vi "MotorenAnsteuern.vi"() -> ()   [LabVIEW 2023]
panel:
  out "IP Adresse":string
  in  "Motor auswählen":string(combo)
  out "Digital":dbl
  out "Drehmoment":dbl
  out "Status/Fehler":dbl
  out "Istgeschwindigkeit":dbl
  out "Handshake":bool
  out "Standby aktiv":bool
  out "Reserviert":bool
  out "SWES inaktiv":bool
  out "Geschwindigkeit erreicht":bool
  out "AS2 aktiv":bool
  out "Warnung":bool
  out "Fehler":bool
  out "in Position":bool
  out "Relativposition übernommen":bool
  out "referenziert":bool
  out "Motor dreht":bool
  out "Bremse geöffnet":bool
  out "Endstufenfreigabe":bool
  out "STO inaktiv":bool
  out "Betriebsbereit":bool
  in  "Stopp":bool
  in  "Digital":dbl
  in  "Deceleration":dbl
  in  "Acceleration":dbl
  in  "Speed":dbl
  in  "Handshake":bool
  in  "Standby":bool
  in  "Inhibit":bool
  in  "Reserviert":bool
  in  "Reservier":bool
  in  "AS2 aktivieren":bool
  in  "Reserviert":bool
  in  "Fehler_Reset":bool
  in  "Start":bool
  in  "Reserviert":bool
  in  "Reserviert":bool
  in  "Reserviert":bool
  in  "Bremse öffnen":bool
  in  "Reserviert":bool
  in  "Enable/ApplicationStop":bool
  in  "Enable/EmergencyStop":bool
  # "zum MOVIDRIVE"
  # "vom MOVIDRIVE"
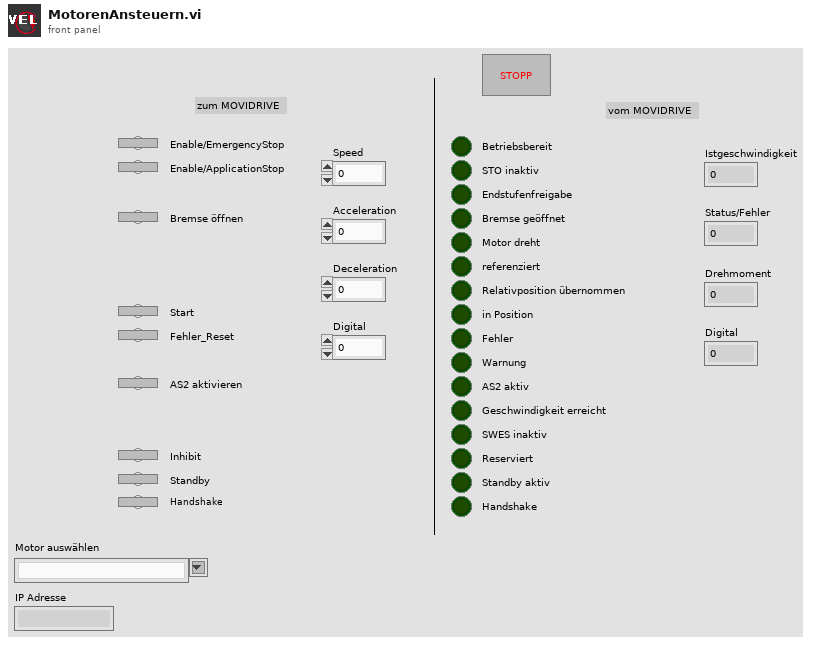
[diagram p1: front panel]
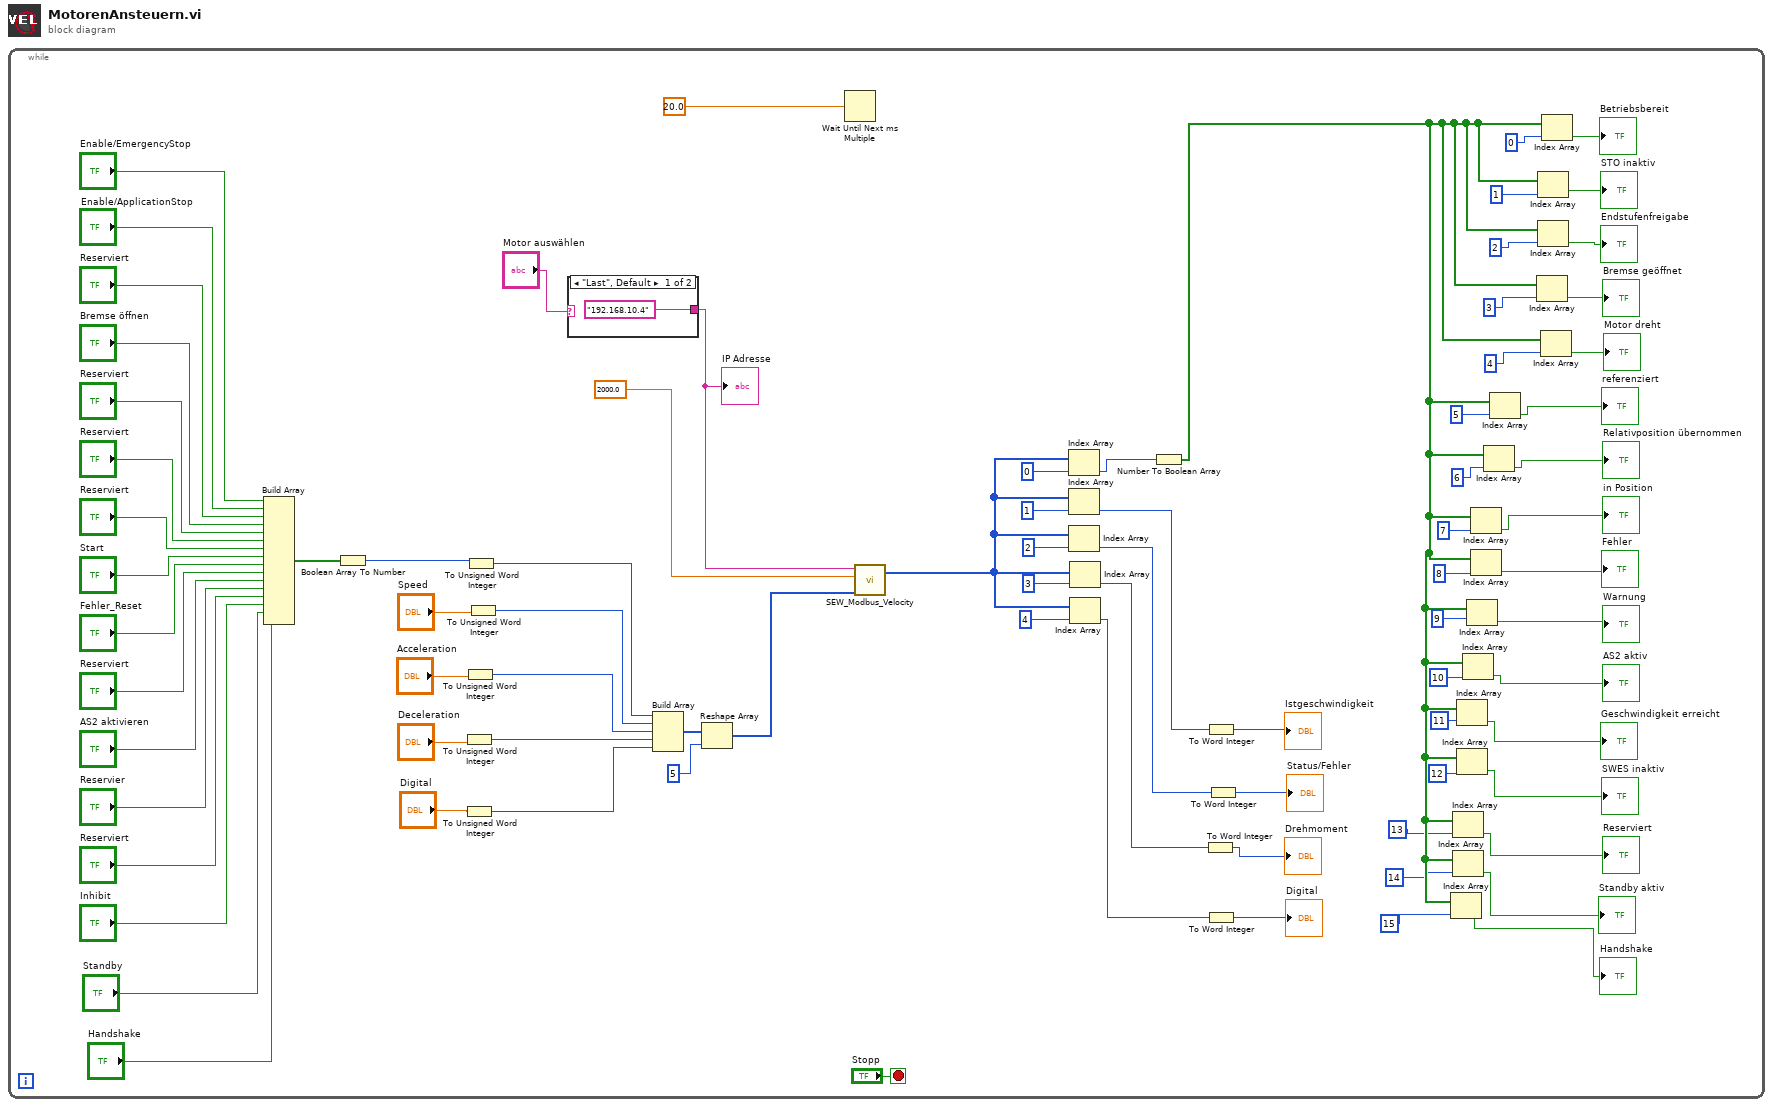
[diagram p0: block diagram]
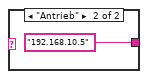
[diagram p2: hidden frame]
diagram:
  n1 = while {
    stop <- "Stopp" stop-if-true
    n2 = Build Array("Enable/EmergencyStop", "Enable/ApplicationStop", "Reserviert", "Bremse öffnen", "Reserviert", "Reserviert", "Reserviert", "Start", "Fehler_Reset", "Reserviert", "AS2 aktivieren", "Reservier", "Reserviert", "Inhibit", "Standby", "Handshake") -> (w71:bool[])
    n3 = Boolean Array To Number(Boolean array=w71) -> (number=w72:u32)
    n4 = To Unsigned Word Integer(number="Deceleration") -> (unsigned 16bit integer=w78:u16)
    n5 = To Unsigned Word Integer(number="Digital") -> (unsigned 16bit integer=w79:u16)
    n6 = To Unsigned Word Integer(number="Acceleration") -> (unsigned 16bit integer=w77:u16)
    n7 = To Unsigned Word Integer(number=w72) -> (unsigned 16bit integer=w76:u16)
    n8 = To Unsigned Word Integer(number="Speed") -> (unsigned 16bit integer=w81:u16)
    n9 = case shown="\"Last\", Default" "Motor auswählen" {
      tunnel: ["192.168.10.4" "192.168.10.5"] -> w1
      frame "Last", Default {
      }
      frame "Antrieb" {
      }
    }
    "IP Adresse" <- w1
    n10 = Build Array(w76, w81, w77, w78, w79) -> (w82:u16[])
    n11 = Reshape Array(w82, 5) -> (w52:u16[])
    n12 = Wait Until Next ms Multiple(millisecond multiple=20.0 ("Update(ms)")) -> ()  [unwired: 1 out]
    n13 = call "SEW_Modbus_Velocity.vi"("Remote IP Address"=w1, "Timeout [ms]"=2000.0 ("Timeout (ms)"), "Output (Write Multiple Register) 2"=w52) -> ("Input (Read Holding Register) 2"=w50:u16[])  [unwired: 3 in]
    n14 = Index Array(array=w50, index=0) -> (element=w36:u16)
    n15 = Index Array(array=w50, index=1) -> (element=w37:u16)
    n16 = Index Array(array=w50, index=2) -> (element=w38:u16)
    n17 = Index Array(array=w50, index=3) -> (element=w39:u16)
    n18 = Index Array(array=w50, index=4) -> (element=w40:u16)
    n19 = Number To Boolean Array(number=w36) -> (Boolean array=w19:bool[])
    n20 = To Word Integer(number=w39) -> (16bit integer=→"Drehmoment":i16)
    n21 = To Word Integer(number=w37) -> (16bit integer=→"Istgeschwindigkeit":i16)
    n22 = To Word Integer(number=w40) -> (16bit integer=→"Digital":i16)
    n23 = To Word Integer(number=w38) -> (16bit integer=→"Status/Fehler":i16)
    n24 = Index Array(array=w19, index=15) -> (element=→"Handshake":bool)
    n25 = Index Array(array=w19, index=13) -> (element=→"Reserviert":bool)
    n26 = Index Array(array=w19, index=14) -> (element=→"Standby aktiv":bool)
    n27 = Index Array(array=w19, index=11) -> (element=→"Geschwindigkeit erreicht":bool)
    n28 = Index Array(array=w19, index=12) -> (element=→"SWES inaktiv":bool)
    n29 = Index Array(array=w19, index=10) -> (element=→"AS2 aktiv":bool)
    n30 = Index Array(array=w19, index=9) -> (element=→"Warnung":bool)
    n31 = Index Array(array=w19, index=7) -> (element=→"in Position":bool)
    n32 = Index Array(array=w19, index=8) -> (element=→"Fehler":bool)
    n33 = Index Array(array=w19, index=6) -> (element=→"Relativposition übernommen":bool)
    n34 = Index Array(array=w19, index=5) -> (element=→"referenziert":bool)
    n35 = Index Array(array=w19, index=3) -> (element=→"Bremse geöffnet":bool)
    n36 = Index Array(array=w19, index=1) -> (element=→"STO inaktiv":bool)
    n37 = Index Array(array=w19, index=2) -> (element=→"Endstufenfreigabe":bool)
    n38 = Index Array(array=w19, index=4) -> (element=→"Motor dreht":bool)
    n39 = Index Array(array=w19, index=0) -> (element=→"Betriebsbereit":bool)
  }
